vi "Create.vi"(8 "error in (no error)":errorcluster, 10 "Comparator":refnum<class "Comparator.lvclass">) -> (0 "error out":errorcluster, 3 "Never Out":refnum<class "Never.lvclass">)   [LabVIEW 2020, in "Never.lvlib" / "Never.lvclass"]
uses:
  Never.lvclass
  Core/Comparator/Comparator.lvclass
  Never.lvclass/Never.ctl
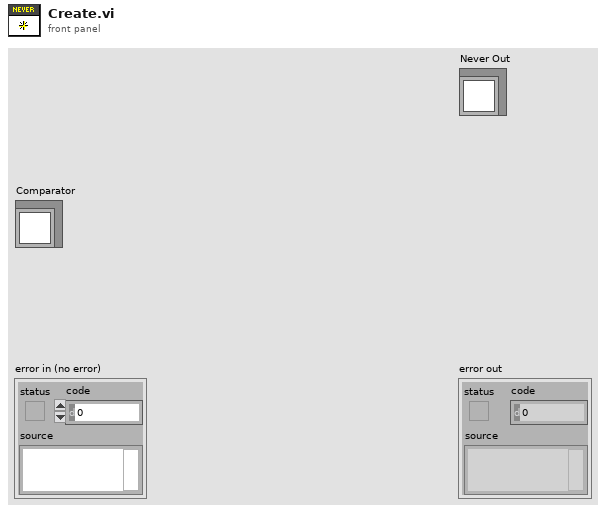
[diagram p1: front panel]
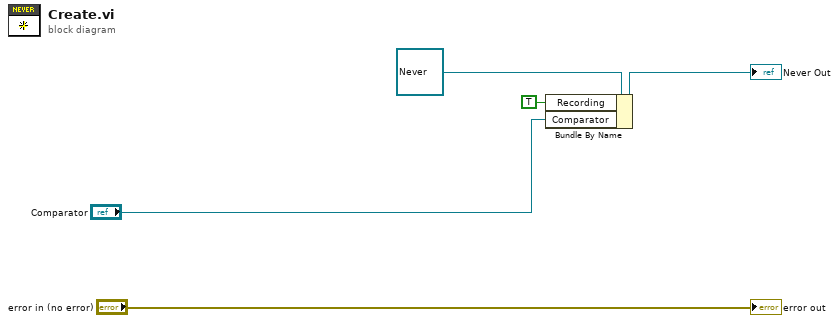
[diagram p0: block diagram]
diagram:
  n1 = Bundle By Name(cluster=refnum<class "Never.lvclass"> refnum ("One"), "Recording"=TRUE, "Comparator"="Comparator") -> (→"Never Out":refnum<class "Never.lvclass">)
  "error out" <- "error in (no error)"
